vi "SMTP Email Send Message Header.vi"(5 "character set":string, 6 "translit":string, 7 "return address":string, 8 "error in (no error)":errorcluster, 9 "recipients":string[](array[string]), 10 "subject":string, 11 "smtp session":T1) -> (0 "error out":errorcluster, 3 "smtp session out":T1)   [LabVIEW 2011, in "NewNI_SMTPEmail.lvlib"]
uses:
  NewNI_SMTPEmail.lvlib
  SMTP Email Session.ctl
panel:
  in  "buffered tcp connection":refnum<k5>
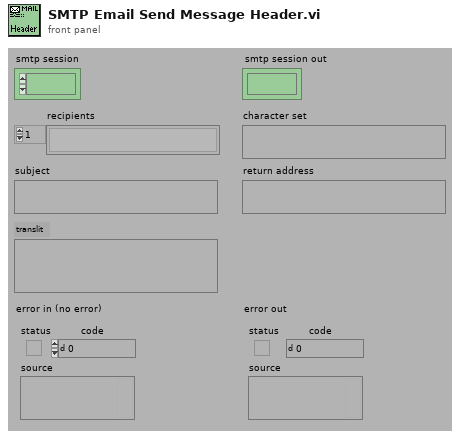
[diagram p1: front panel]
types:
  T1 = typedef "NewNI_SMTPEmail.lvlib/SMTP Email Session.ctl" = refnum<k1>
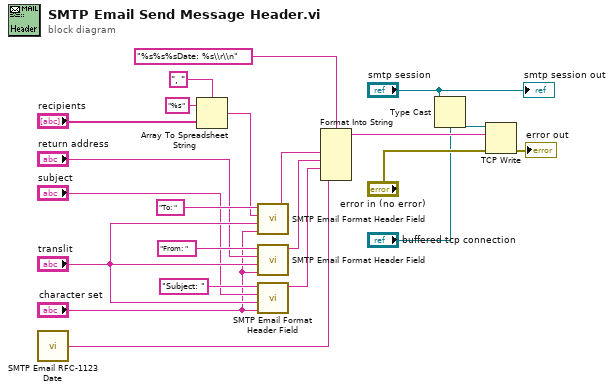
[diagram p0: block diagram]
diagram:
  n1 = call "SMTP Email RFC-1123 Date.vi"() -> ("GMT Date/Time"=w8:string)  [unwired: 1 in, 1 out]
  n2 = Array To Spreadsheet String(delimiter (Tab)=", ", array="recipients", 3:"%s" ("format string")) -> (spreadsheet string=w7:string)
  n3 = call "SMTP Email Format Header Field.vi"("character set"="character set", "translit"="translit", "header content"=w7, "header name (Subject: )"="To: " ("subject out")) -> ("encoded header line"=w6:string)  [unwired: 1 in, 2 out]
  n4 = call "SMTP Email Format Header Field.vi"("character set"="character set", "translit"="translit", "header content"="return address", "header name (Subject: )"="From: " ("subject out")) -> ("encoded header line"=w13:string)  [unwired: 1 in, 2 out]
  n5 = call "SMTP Email Format Header Field.vi"("character set"="character set", "translit"="translit", "header content"="subject", "header name (Subject: )"="Subject: " ("subject out")) -> ("encoded header line"=w1:string)  [unwired: 1 in, 2 out]
  n6 = Format Into String(format string="%s%s%sDate: %s\\r\\n", w6, w13, w1, w8) -> (resulting string=w19:string)  [unwired: 2 in, 1 out]
  n7 = Type Cast(type="buffered tcp connection", x="smtp session") -> (*(type *) &x=w16:refnum<k5>)
  n8 = TCP Write(connection ID=w16, data in=w19, error in (no error)="error in (no error)") -> (error out=→"error out":errorcluster)  [unwired: 3 out]
  "smtp session out" <- "smtp session"
